vi "overall tab1.vi"() -> ()   [LabVIEW 2020]
panel:
  in  "Tab Control":enum32{"Add 1 digit number", "Add Mix number"}(tab)
  out "A + B 4":string
  out "B":string
  out "A":string
  out "A + B":dbl
  in  "B":dbl
  in  "A":dbl
  out "A":bool[](array[boolean])
  out "B":bool[](array[boolean])
  out "A + B":bool[][](array[boolean])
  out "A + B":string
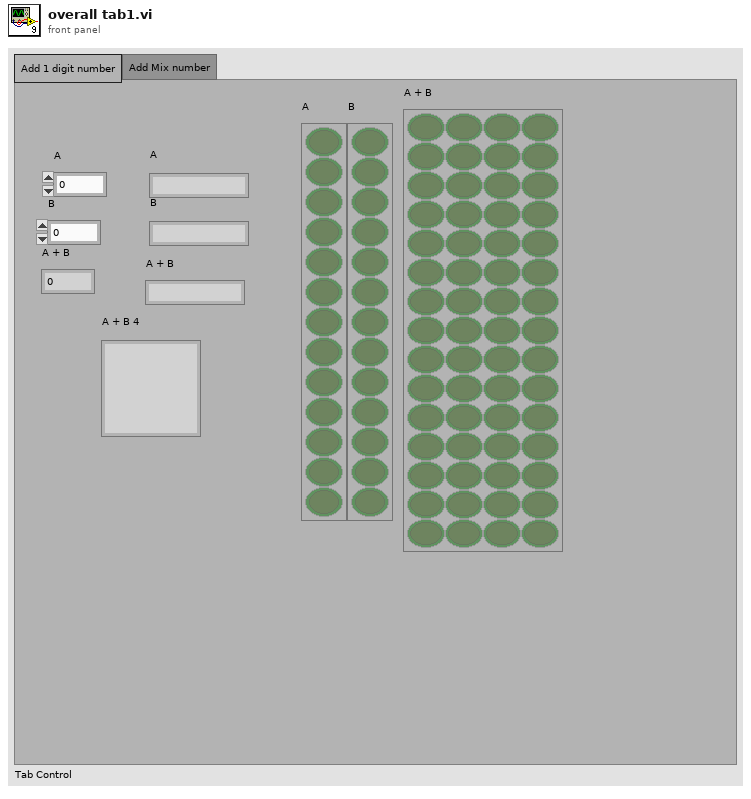
[diagram p1: front panel]
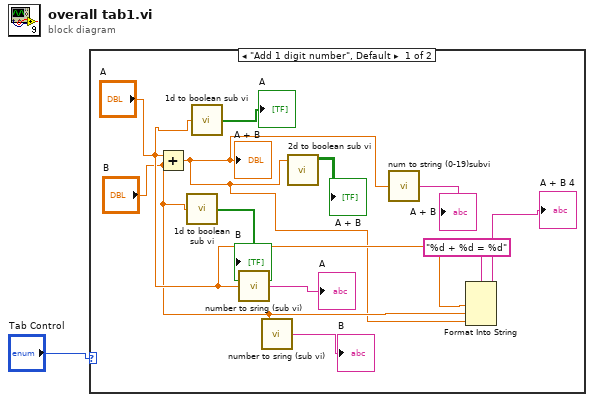
[diagram p0: block diagram]
diagram:
  n1 = case shown="\"Add 1 digit number\", Default" "Tab Control" {
    frame "Add 1 digit number", Default {
      n2 = Add(x="A", y="B") -> (x+y=w9:dbl)
      "A + B" <- w9
      n3 = call "1d to boolean sub vi.vi"("A"="B") -> ("initialized array"=→"B":bool[])
      n4 = call "1d to boolean sub vi.vi"("A"="A") -> ("initialized array"=→"A":bool[])
      n5 = call "number to sring (sub vi).vi"("Numeric"="A") -> ("element"=→"A":string)
      n6 = call "number to sring (sub vi).vi"("Numeric"="B") -> ("element"=→"B":string)
      n7 = call "2d to boolean sub vi.vi"("Numeric"=w9) -> ("initialized array"=→"A + B":bool[][])  [unwired: 10 in]
      n8 = call "num to string (0-19)subvi.vi"("Numeric"=w9) -> ("element"=→"A + B":string)
      n9 = Format Into String "Format Into String"(format string="%d + %d = %d", "A", "B", w9) -> (resulting string=→"A + B 4":string)  [unwired: 2 in, 1 out]
    }
    frame "Add Mix number" {
    }
  }
